vi "2_AM.vi"() -> ()   [LabVIEW 2026]
uses:
  <vilib>/measure/maresamp.llb/Align M + N Waveforms (single shot).vi
  <vilib>/measure/NI_MAPro.lvlib
panel:
  out "Filtered Signal":dynamicdata(graph)
  out "Waveform Graph":waveform(dbl)[](graph)
  out "message":dynamicdata(graph)
  out "carrier":dynamicdata(graph)
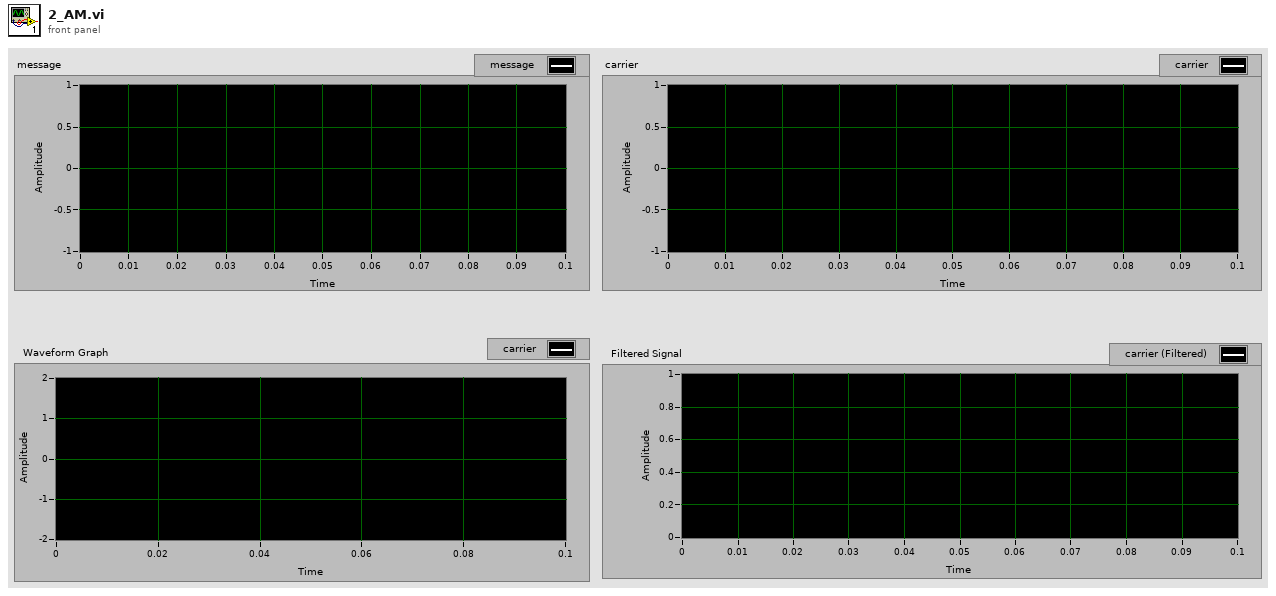
[diagram p1: front panel]
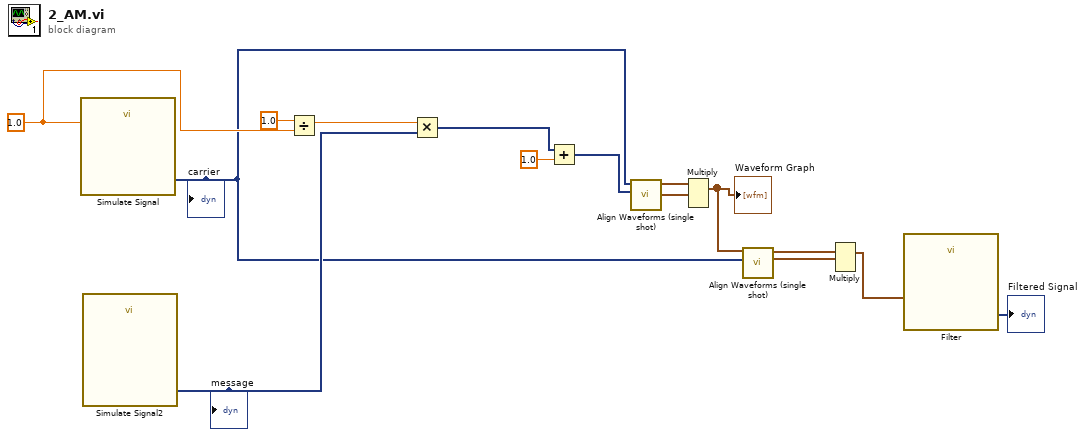
[diagram p0: block diagram]
diagram:
  w15 = 1.0 ("Amplitude")
  n1 = call "Simulate Signal"("Amplitude"=w15) -> ("carrier"=w5:dynamicdata)  [unwired: 13 in, 1 out]
  "carrier" <- w5
  n2 = call "Simulate Signal2"() -> ("message"=w12:dynamicdata)  [unwired: 14 in, 1 out]
  "message" <- w12
  n3 = Divide(x=1.0, y=w15) -> (x/y=w13:dbl)
  n4 = Multiply(x=w13, y=w12) -> (x*y=w11:dynamicdata)
  n5 = Add(x=w11, y=1.0) -> (x+y=w9:dynamicdata)
  n6 = call-poly <vilib>:"Align Waveforms (single shot).vi"("N waveforms in"=w9, "M waveforms in"=w5) -> ("N aligned waveforms out"=w7:waveform(dbl)[], "M aligned waveforms out"=w8:waveform(dbl)[])  [unwired: 7 in, 1 out]
  n7 = Multiply(1:w7, 2:w8) -> (0:w6:waveform(dbl)[])  [unwired: 1 in, 1 out]
  "Waveform Graph" <- w6
  n8 = call-poly <vilib>:"Align Waveforms (single shot).vi"("N waveforms in"=w5, "M waveforms in"=w6) -> ("N aligned waveforms out"=w3:waveform(dbl)[], "M aligned waveforms out"=w4:waveform(dbl)[])  [unwired: 7 in, 1 out]
  n9 = Multiply(1:w3, 2:w4) -> (0:w2:waveform(dbl)[])  [unwired: 1 in, 1 out]
  n10 = call "Filter"("Signal"=w2) -> ("Filtered Signal"=→"Filtered Signal":dynamicdata)  [unwired: 9 in, 1 out]
